vi "Write Carrier frequency.vi"(8 "error in (no error)":errorcluster, 10 "Carrier frequency":dbl(knob)=440.0 scale=0.0..1000.0, 11 "HRF_Device in":refnum<class "HRF_Device.lvclass">) -> (0 "error out":errorcluster, 3 "HRF_Device out":refnum<class "HRF_Device.lvclass">)   [LabVIEW 2020, in "HRF_Device.lvclass"]
uses:
  HRF_Device.lvclass
  HRF_Device.lvclass/HRF_Device.ctl
  D:/work/HackRF/Labview Driver/NetHackrf.dll
  NetHackrf.dll
  Read Device ref.vi
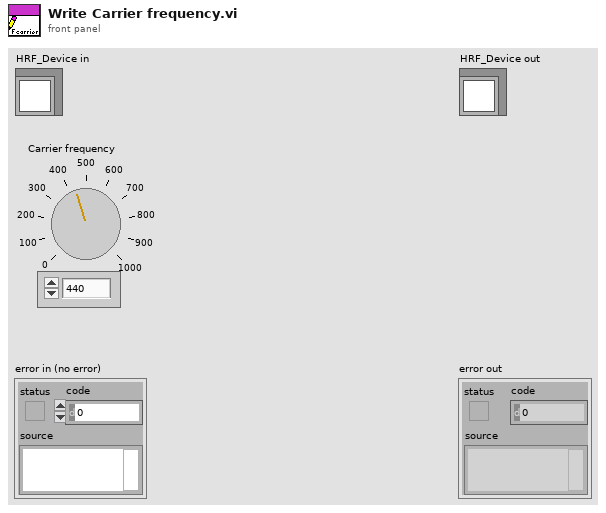
[diagram p1: front panel]
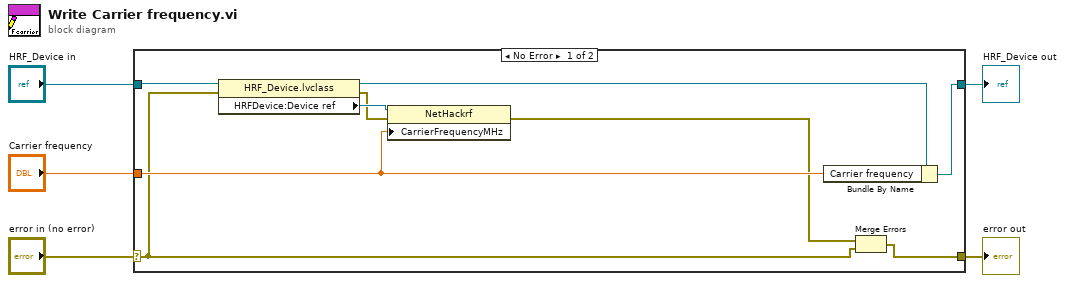
[diagram p0: block diagram]
diagram:
  n1 = case shown="No Error" "error in (no error)" {
    selector: "error in (no error)" -> [w8 w15]
    tunnel: [w7 w15] -> w4
    tunnel: [w14 w16] -> w2
    tunnel: "HRF_Device in" -> [w11 w16]
    tunnel: "Carrier frequency" -> [w9 _]
    frame No Error {
      n2 = property class="HRF_Device.lvclass"(reference=w11, error in=w8) -> (reference out=w10:refnum<class "HRF_Device.lvclass">, error out=w12:errorcluster, "HRFDevice:Device ref"=w13:refnum<k24>)
      n3 = property class="NetHackrf"(reference=w13, error in=w12, "CarrierFrequencyMHz"=w9) -> (error out=w6:errorcluster)  [unwired: 1 out]
      n4 = Bundle By Name(cluster=w10, "Carrier frequency"=w9) -> (w14:refnum<class "HRF_Device.lvclass">)
      n5 = Merge Errors(w6, w8) -> (w7:errorcluster)
    }
    frame Error {
    }
  }
  "error out" <- w4
  "HRF_Device out" <- w2
